vi "Update.vi"(8 "error in (no error)":errorcluster, 11 "PredictiveMaintenance in":refnum<class "PredictiveMaintenance.lvclass">) -> (0 "error out":errorcluster, 3 "PredictiveMaintenance out":refnum<class "PredictiveMaintenance.lvclass">)   [LabVIEW 2019, in "PredictiveMaintenance.lvlib" / "PredictiveMaintenance.lvclass"]
uses:
  PredictiveMaintenance.lvclass
  PredictiveMaintenance.lvclass/PredictiveMaintenance.ctl
  typedefs/Trigger_Data.ctl
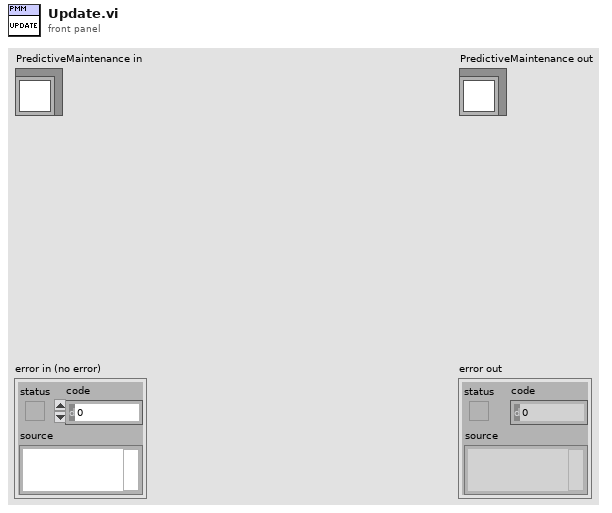
[diagram p1: front panel]
types:
  T1 = typedef "PredictiveMaintenance.lvlib/PredictiveMaintenance.lvclass/Trigger_Data.ctl" = cluster{"trigger":string, "curr_val (h)":dbl, "warn_limit (h)":dbl, "err_limit (h)":dbl, "running_timestamp":timestamp, "counter (h)":dbl}
  T2 = typedef "PredictiveMaintenance.lvlib/PredictiveMaintenance.lvclass/UI_Control.ctl" = cluster{"String":string, "slider":dbl, "slider_background":cluster{"Numeric":dbl, "Numeric":dbl, "Numeric":dbl}, "curr_value":dbl, "warn_value":dbl, "err_value":dbl, "colorbox":u32}
  T3 = typedef "PredictiveMaintenance.lvlib/PredictiveMaintenance.lvclass/EventData.ctl" = cluster{"event":string, "curr_val":dbl, "warn_limit":dbl, "err_limit":dbl}
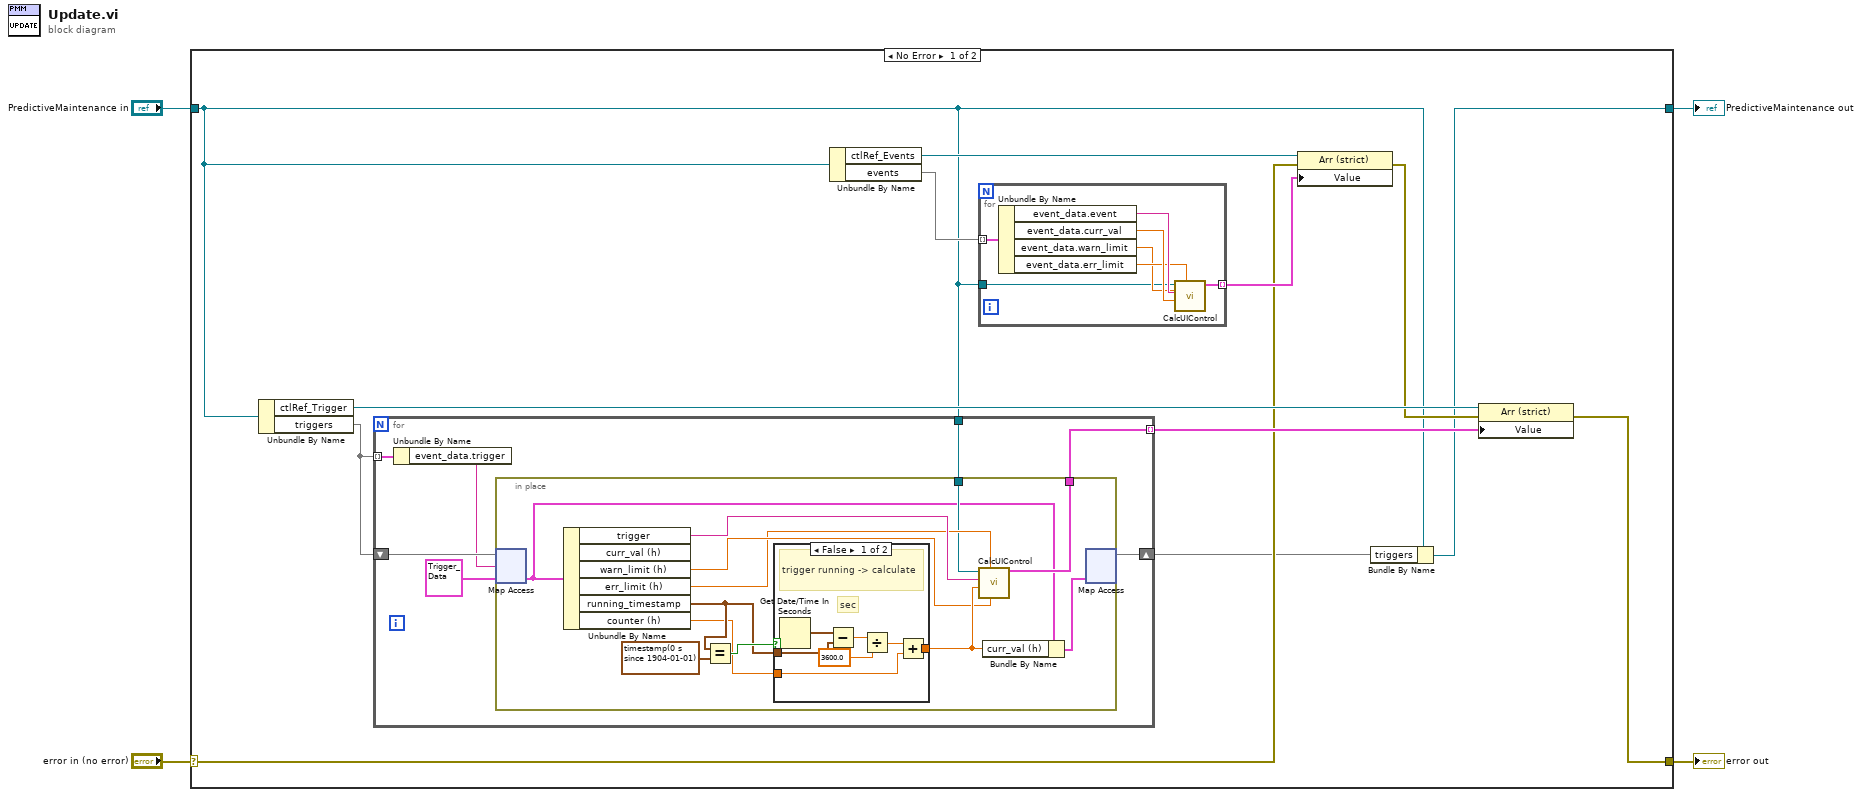
[diagram p0: block diagram]
diagram:
  n1 = case shown="No Error" "error in (no error)" {
    selector: "error in (no error)" -> [w10 w52]
    tunnel: [w5 w52] -> w3
    tunnel: [w6 w51] -> w1
    tunnel: "PredictiveMaintenance in" -> [w9 w51]
    frame No Error {
      n2 = Unbundle By Name(w9) -> ("ctlRef_Trigger"=w13:refnum<vi>, "triggers"=w8:map{string, T1})
      n3 = for {
        tunnel: w8 -> [w26] mode=indexing
        tunnel: w9 -> [w29]
        tunnel: [w28] -> w12 mode=indexing
        shift-right: [w27] -> w7
        shift-left: w8 -> [w30]
        n4 = Unbundle By Name(w26) -> ("event_data.trigger"=w25:string)
        n5 = in-place {
          in-place-border: w29 -> [w35]
          in-place-border: [w33] -> w28
          n6 = in-place-map #1(w30, w25, T1 {"trigger"="", "curr_val (h)"=0.0, "warn_limit (h)"=0.0, "err_limit (h)"=0.0, "running_timestamp"=timestamp(0 s since 1904-01-01), "counter (h)"=0.0} ("event_data")) -> (w32:T1)  [unwired: 1 out]
          n7 = Unbundle By Name(w32) -> ("trigger"=w41:string, "warn_limit (h)"=w40:dbl, "err_limit (h)"=w39:dbl, "running_timestamp"=w37:timestamp, "counter (h)"=w36:dbl)  [unwired: 1 out]
          n8 = Equal?(x=w37, y=timestamp(0 s since 1904-01-01) ("event_data.running_timestamp")) -> (x = y?=w38:bool)
          n9 = case shown="False" w38 {
            tunnel: w37 -> [w48 _]
            tunnel: [w44 w50] -> w42
            tunnel: w36 -> [w43 w50]
            frame False {
              # "sec"
              # "trigger running -> calculate"
              n10 = Get Date/Time In Seconds() -> (seconds since 1Jan1904=w49:timestamp)
              n11 = Subtract(x=w49, y=w48) -> (x-y=w47:dbl)
              n12 = Divide(x=w47, y=3600.0) -> (x/y=w45:dbl)
              n13 = Add(x=w45, y=w43) -> (x+y=w44:dbl)
            }
            frame True {
              # "trigger stopped or never running"
            }
          }
          n14 = call "CalcUIControl.vi"("warn_limit"=w40, "err_limit"=w39, "curr_val"=w42, "event"=w41, "PredictiveMaintenance in"=w35) -> ("UICtrl_Data"=w33:T2)  [unwired: 6 in]
          n15 = Bundle By Name(cluster=w32, "curr_val (h)"=w42) -> (w31:T1)
          n16 = in-place-map #1(w31) -> (w27:map{string, T1})  [unwired: 1 in, 2 out]
        }
      }
      n17 = Unbundle By Name(w9) -> ("ctlRef_Events"=w16:refnum<vi>, "events"=w15:map{string, T3})
      n18 = for {
        tunnel: w15 -> [w23] mode=indexing
        tunnel: [w21] -> w14 mode=indexing
        tunnel: w9 -> [w17]
        n19 = Unbundle By Name(w23) -> ("event_data.event"=w22:string, "event_data.curr_val"=w20:dbl, "event_data.warn_limit"=w18:dbl, "event_data.err_limit"=w19:dbl)
        n20 = call "CalcUIControl.vi"("warn_limit"=w18, "err_limit"=w19, "curr_val"=w20, "event"=w22, "PredictiveMaintenance in"=w17) -> ("UICtrl_Data"=w21:T2)  [unwired: 6 in]
      }
      n21 = property class="Arr (strict)"(reference=w16, error in=w10, "Value"=w14) -> (error out=w11:errorcluster)  [unwired: 1 out]
      n22 = Bundle By Name(cluster=w9, "triggers"=w7) -> (w6:refnum<class "PredictiveMaintenance.lvclass">)
      n23 = property class="Arr (strict)"(reference=w13, error in=w11, "Value"=w12) -> (error out=w5:errorcluster)  [unwired: 1 out]
    }
    frame Error {
    }
  }
  "error out" <- w3
  "PredictiveMaintenance out" <- w1
